vi "A2_Maquina_Estados02.vi"() -> ()   [LabVIEW 2025]
panel:
  out "Estado 02":bool
  out "Estado 01":bool
  out "Estado por defecto":bool
  in  "stop":bool
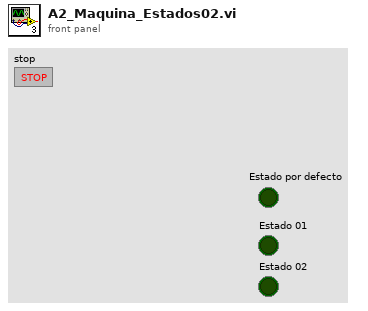
[diagram p1: front panel]
types:
  T1 = enum16{"Estado Defecto", "Estado 01", "Estado 02", "Estado 03"}
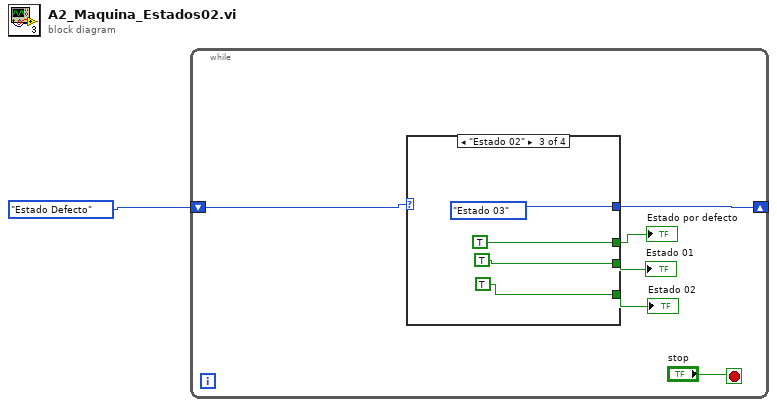
[diagram p0: block diagram]
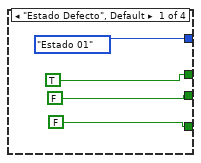
[diagram p2: hidden frame]
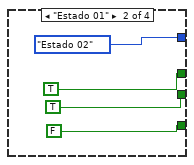
[diagram p3: hidden frame]
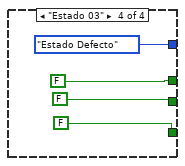
[diagram p4: hidden frame]
diagram:
  n1 = while {
    shift-right: [w6] -> _
    shift-left: T1."Estado Defecto" -> [w5]
    stop <- "stop" stop-if-true
    n2 = case shown="\"Estado 02\"" w5 {
      tunnel: [T1."Estado 01" T1."Estado 02" T1."Estado 03" T1."Estado Defecto"] -> w6
      tunnel: [TRUE TRUE TRUE FALSE] -> w4
      tunnel: [FALSE TRUE TRUE FALSE] -> w3
      tunnel: [FALSE FALSE TRUE FALSE] -> w2
      frame "Estado Defecto", Default {
      }
      frame "Estado 01" {
      }
      frame "Estado 02" {
      }
      frame "Estado 03" {
      }
    }
    "Estado 01" <- w3
    "Estado 02" <- w2
    "Estado por defecto" <- w4
  }
